vi "analyze-z-axis.vi"() -> ()   [LabVIEW 2015]
uses:
  <vilib>/rvi/Emulation/niFpgaGetClockAttributes.vi
  <vilib>/rvi/Emulation/niFpgaSctlEmulationGetInTimedLoop.vi
  <vilib>/rvi/Emulation/niFpgaEmulationReportErrorSimple.vi
  <vilib>/rvi/eio/common/nirviEmuTemplateMethod_errors.vi
  <vilib>/rvi/Emulation/niFpgaEmulationIsFPGAContextNoSignature.vi
  <vilib>/rvi/DataTransferAndStorage/Container/Common/niFpgaContainerGetUniqueNameForEmu.vi
  <vilib>/rvi/Memory/Memory_Emulation/niFpgaMemoryEmulationCacheClearOnFirstRun.vi
  <vilib>/rvi/Memory/Memory_Emulation/nirvimemoryEmulationManagerCache_MakeExclusive.vi
  <vilib>/rvi/Memory/Memory_Emulation/niFpgaMemoryEmulationValidateCache.vi
  <vilib>/rvi/Memory/Memory_Emulation/nirvimemoryEmulationManagerCache_InsertValue.vi
  <vilib>/Utility/error.llb/Clear Errors.vi
  <vilib>/rvi/Memory/Memory_Emulation/nirvimemoryEmulationManagerCache_ReleaseExclusive.vi
  <vilib>/rvi/Memory/Memory_Emulation/nirvimemoryEmulationManagerCache_GetValue.vi
  <vilib>/rvi/Memory/Memory_Emulation/nirvimemoryEmulationManagerCache_SetValue.vi
  <vilib>/rvi/Emulation/niFpgaProcessEmulError.vi
  <vilib>/rvi/DataTransferAndStorage/Container/Common/niFpgaContainerExecOnDevCompGetState.vi
  <vilib>/rvi/errors/niFpgaSetErrorForExecOnDevCompSimple.vi
  <vilib>/rvi/eio/common/nirviEmuReportErrorAndStop.vi
  <vilib>/rvi/FIFO/Fifo_Resource/nirvififoEmulationSetSize.vi
  <vilib>/rvi/FIFO/Fifo_Resource/nirviFifoEmulationQueueMgr.vi
  <instcachedir>/0/nirviFifoEmulationQueueMgr_E5CAEC123FF24DC58D834DCA3CDAA9B5.lvgen/nirviFifoEmulationQueueMgr_E5CAEC123FF24DC58D834DCA3CDAA9B5_003.vi
  <vilib>/rvi/FIFO/Fifo_Resource/nirvififoEmulationDetermineInputValidOut.vi
  <vilib>/rvi/FIFO/Fifo_Resource/nirvififoEmulationCreateLock.vi
  <vilib>/rvi/FIFO/Fifo_Resource/nirvififoEmulationObtainLock.vi
  <vilib>/rvi/FIFO/Fifo_Resource/nirvififoEmulationReleaseLock.vi
  <vilib>/rvi/occurrence/nirviWaitOnOccurrenceBase.vi
  <vilib>/rvi/errors/nirviReportUnexpectedCaseInternalError.vi
  <vilib>/rvi/errors/nirviReportUnexpectedCaseInternalError (U32).vi
  <vilib>/rvi/interface/RandomDataEmulation/niFpgaRandomDataHandleErrors.vi
  <vilib>/rvi/Emulation/niFpgaCriticalErrorInLSC.vi
  <vilib>/eio/EIONode/EIONode.xnode
  <vilib>/rvi/DataTransferAndStorage/Container/XNode/niFpgaContainer.xnode
  <vilib>/rvi/DataTransferAndStorage/Register/Emulation/niFpgaRegisterEmulation.vi
  <vilib>/rvi/FIFO/Fifo_Resource/niFpgaFifoEmulationRefIn.vi
  libimaging-cs.lvlib
panel:
  in  "stop":bool
  out "caseiter":i16
  out "currentCase":i16
  in  "uz-max":sgl
  in  "numIters":i16
  out "u(k)":sgl
  in  "ramp-rate":sgl format="%#_13g"
  in  "TOL":sgl format="%#_13g"
  in  "init Z up":sgl
  in  "trigger-0":bool
  out "Mod2/AI2":fxp<+/-,24,5>
  in  "initial-case":u8
  in  "Ki":sgl format="%#_13g"
  in  "setpoint":sgl format="%#_13g"
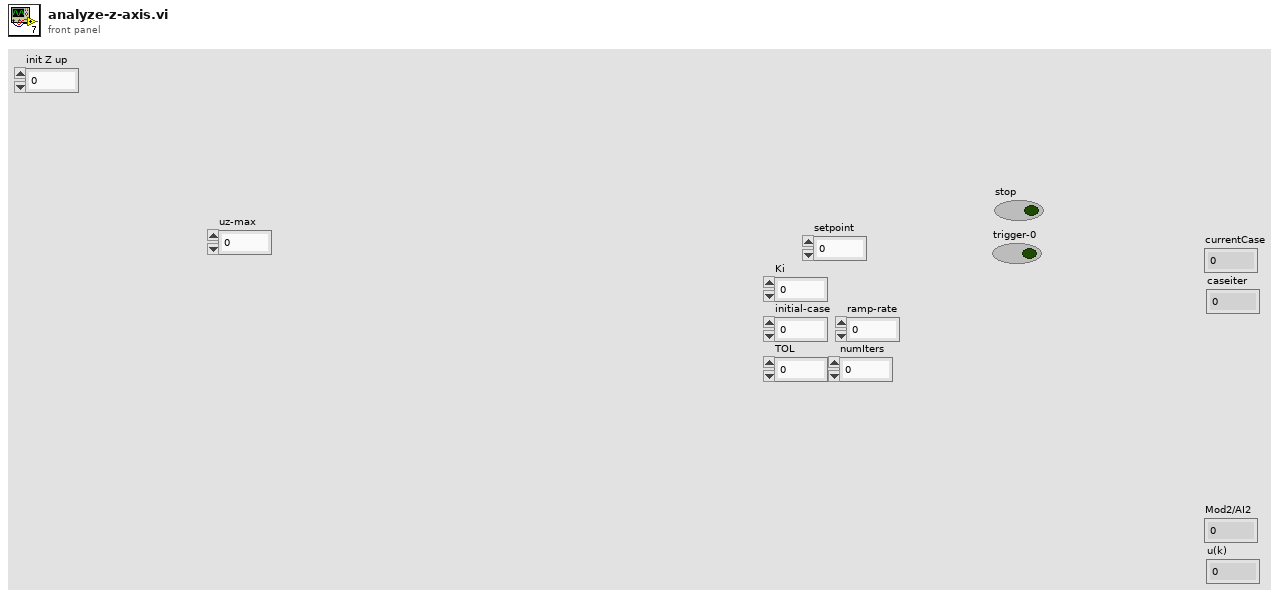
[diagram p1: front panel]
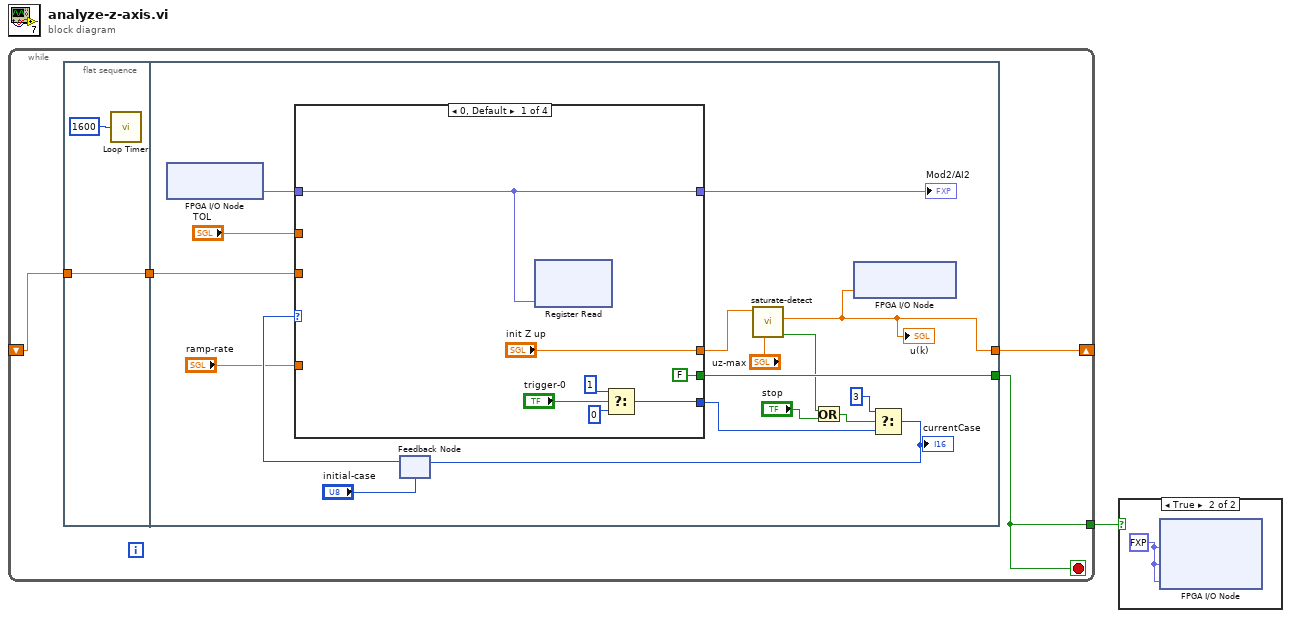
[diagram p0: block diagram]
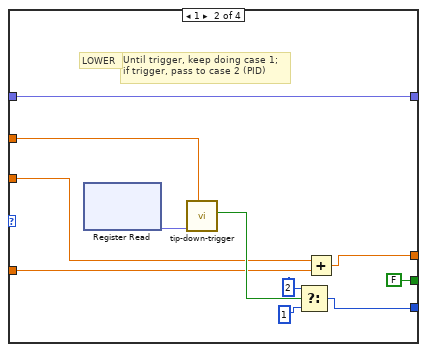
[diagram p3: hidden frame]
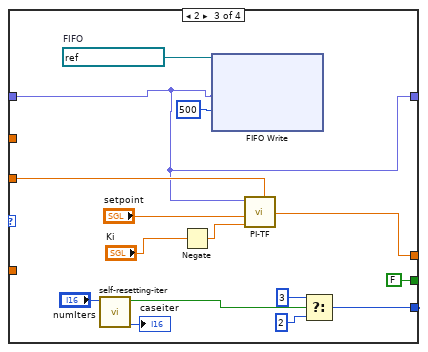
[diagram p4: hidden frame]
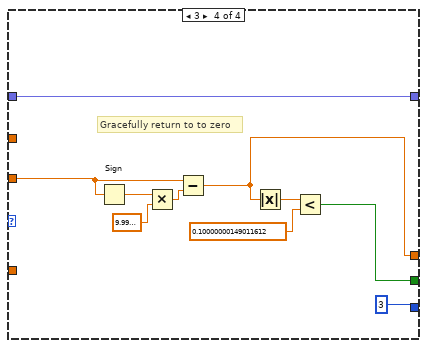
[diagram p5: hidden frame]
diagram:
  n1 = while {
    shift-right: [w5] -> _
    shift-left: _ -> [w3]
    tunnel: [w2] -> w1
    stop <- w2 stop-if-true
    n2 = flat-sequence {
      tunnel: w3 -> [w6]
      tunnel: [w6] -> w4
      tunnel: [w9] -> w5
      tunnel: w4 -> [w24]
      tunnel: [w18] -> w2
      frame #0 {
        n3 = call "Loop Timer"("Count(Ticks)"=u32 1600) -> ()  [unwired: 1 out]
      }
      frame #1 {
        n4 = xnode "FPGA I/O Node"() -> ("Mod2/AI2"=w21:fxp<+/-,24,5>)  [unwired: 1 in, 1 out]
        n5 = feedback #1("initial-case") -> (w23:i16)
        n6 = case shown="0, Default" w23 {
          tunnel: ["init Z up" w37 w54 w61] -> w12
          tunnel: w24 -> [_ w35 w53 w62]
          tunnel: [w26 w36 w47 i16 3 ("t")] -> w16
          tunnel: w21 -> [w28 w42 w44 w60]
          tunnel: [w28 w42 w44 w60] -> w20
          tunnel: "ramp-rate" -> [_ w34 _ _]
          tunnel: [FALSE FALSE FALSE w59] -> w18
          tunnel: "TOL" -> [_ w32 _ _]
          frame 0, Default {
            n7 = xnode ("Register Read")("Data"=w28) -> ()  [unwired: 1 in, 1 out]
            n8 = Select(t=i16 1, s="trigger-0", f=i16 0) -> (s? t:f=w26:i16)
          }
          frame 1 {
            # "Until trigger, keep doing case 1;\nif trigger, pass to case 2 (PID)"
            # "LOWER"
            n9 = xnode ("Register Read")() -> ("Data"=w39:fxp<+/-,16,5>)  [unwired: 1 in, 1 out]
            n10 = call "tip-down-trigger.vi"("TOL"=w32, "Vo"=w39) -> ("trigger"=w38:bool)  [unwired: 9 in]
            n11 = Select(t=i16 2, s=w38, f=i16 1) -> (s? t:f=w36:i16)
            n12 = Add(x=w35, y=w34) -> (x+y=w37:sgl)
          }
          frame 2 {
            w57 = refnum<k21> "fpga-to-host2"  # FIFO
            n13 = call "self-resetting-iter.vi"("zup-N"="numIters") -> ("Numeric"=→"caseiter":i16, "Boolean"=w49:bool)  [unwired: 9 in]
            n14 = Negate(x="Ki") -> (-x=w52:sgl)
            n15 = xnode ("FIFO Write")("Element"=w44, "Timeout"=500, "FIFO In"=w57) -> ()  [unwired: 2 out]
            n16 = call "PI-TF.vi"("u(k-1)"=w53, "Ki"=w52, "setpoint"="setpoint", "y(k)"=w44) -> ("u(k)"=w54:sgl)  [unwired: 7 in]
            n17 = Select(t=i16 3, s=w49, f=i16 2) -> (s? t:f=w47:i16)
          }
          frame 3 {
            # "Gracefully return to to zero"
            n18 = Sign(1:w62) -> (0:w67:sgl)
            n19 = Multiply(x=w67, y=sgl 1e-05) -> (x*y=w66:sgl)
            n20 = Subtract(x=w62, y=w66) -> (x-y=w61:sgl)
            n21 = Absolute Value(x=w61) -> (abs(x)=w65:sgl)
            n22 = Less?(x=w65, y=sgl 0.1) -> (x < y?=w59:bool)
          }
        }
        "Mod2/AI2" <- w20
        n23 = call "saturate-detect.vi"("bound"="uz-max", "x"=w12) -> ("saturated"=w11:bool, "sat(x)"=w9:sgl)  [unwired: 8 in]
        "u(k)" <- w9
        n24 = Or(x=w11, y="stop") -> (x .or. y?=w10:bool)
        n25 = xnode "FPGA I/O Node"("Mod1/AO2"=w9) -> ()  [unwired: 1 in, 1 out]
        n26 = Select(t=i16 3, s=w10, f=w16) -> (s? t:f=w17:i16)
        "currentCase" <- w17
        n27 = feedback-in #1(w17) -> ()
      }
    }
  }
  n28 = case shown="True" w1 {
    frame False {
    }
    frame True {
      w68 = fxp<+,1,1> 0.0
      n29 = xnode "FPGA I/O Node"("Mod1/AO0"=w68, "Mod1/AO1"=w68, "Mod1/AO2"=w68) -> ()  [unwired: 3 in, 3 out]
    }
  }
